vi "FormatCommand.vi"(7 "CMD (MON)":u8(ring) items=["MON", "SET"], 8 "VAL":string, 9 "PAR":string(combo)="BDNAME", 10 "CH":i8=-1 min=-1 max=4, 11 "BD (0)":u8 max=31) -> (3 "cmd":string)   [LabVIEW 2018, in "CAEN PSM.lvlib"]
uses:
  <instrlib>/CAEN PSM/CAEN PSM.lvlib
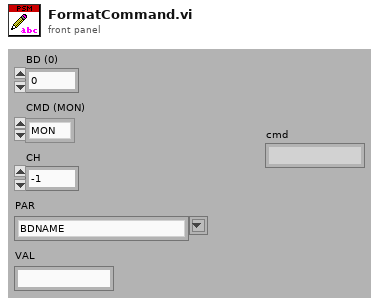
[diagram p1: front panel]
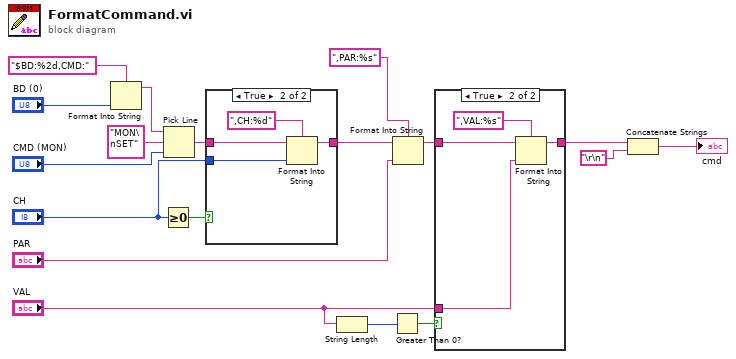
[diagram p0: block diagram]
diagram:
  n1 = Format Into String(format string="$BD:%2d,CMD:", "BD (0)") -> (resulting string=w14:string)  [unwired: 2 in, 1 out]
  n2 = Greater Or Equal To 0?(x="CH") -> (x >= 0?=w13:bool)
  n3 = Pick Line(string ("")=w14, multi-line string="MON\nSET", line index="CMD (MON)") -> (output string=w11:string)
  n4 = case shown="True" w13 {
    tunnel: "CH" -> [_ w22]
    tunnel: w11 -> [w19 w21]
    tunnel: [w19 w20] -> w6
    frame False {
    }
    frame True {
      n5 = Format Into String(format string=",CH:%d", initial string=w21, w22) -> (resulting string=w20:string)  [unwired: 1 in, 1 out]
    }
  }
  n6 = String Length(string="VAL") -> (length=w10:i32)
  n7 = Greater Than 0?(x=w10) -> (x > 0?=w9:bool)
  n8 = Format Into String(format string=",PAR:%s", initial string=w6, "PAR") -> (resulting string=w4:string)  [unwired: 1 in, 1 out]
  n9 = case shown="True" w9 {
    tunnel: "VAL" -> [_ w27]
    tunnel: [w24 w26] -> w2
    tunnel: w4 -> [w24 w25]
    frame False {
    }
    frame True {
      n10 = Format Into String(format string=",VAL:%s", initial string=w25, w27) -> (resulting string=w26:string)  [unwired: 1 in, 1 out]
    }
  }
  n11 = Concatenate Strings(w2, "\r\n") -> (→"cmd":string)
